vi "DataFinder Invoke Node.vi"   [LabVIEW 2020]
doc: "Provides methods that you use to configure the DataFinder."
uses:
  <resource>/objmgr/DataFinder.rc
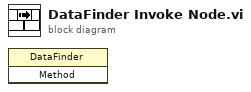
[diagram p0: block diagram]
diagram:
  n1 = invoke class="DataFinder" method=#-1() -> ()  [unwired: 3 in, 3 out]
